vi "notifier.vi"() -> ()   [LabVIEW 2013]
panel:
  out "notifier":refnum<notifier>
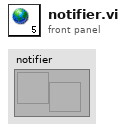
[diagram p1: front panel]
diagram:
